vi "pH theoretical.vi"(2 "pH cal":dbl=7.0 format="%.2f", 3 "V/T cal":dbl format="%.5f", 5 "V/T":dbl format="%.5f") -> (1 "Theoretical pH":dbl format="%.2f")   [LabVIEW 2012]
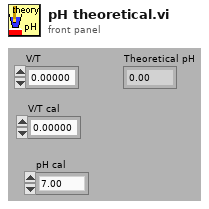
[diagram p1: front panel]
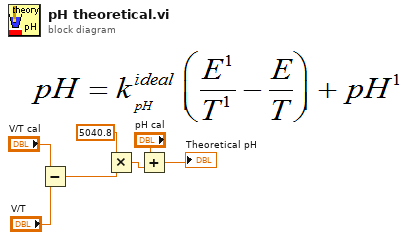
[diagram p0: block diagram]
diagram:
  n1 = Subtract(x="V/T cal", y="V/T") -> (x-y=w4:dbl)
  n2 = Multiply(x=5040.8, y=w4) -> (x*y=w3:dbl)
  n3 = Add(x="pH cal", y=w3) -> (x+y=→"Theoretical pH":dbl)
